vi "Begin.vi"() -> (0 "error out":errorcluster)   [LabVIEW 2011]
doc: "Called before other user functions, this VI is expected to open initial I/O refnums, load in file data, and do all program initialization. Notice that the <B>error out</B> terminal is simply used for data flow. Wiring it to other structures or subVIs ensures that this VI runs first."
uses:
  <vilib>/Rock Robotics/WPI/Joystick/WPI_JoystickDeviceEnum.ctl
  <vilib>/Rock Robotics/SystemInterfaces/AI/FPGA_AIChannel.ctl
  <vilib>/Rock Robotics/SystemInterfaces/Typedef/FPGA_TypedefAnalogModule.ctl
  <vilib>/Rock Robotics/SystemInterfaces/Typedef/FPGA_TypedefDigitalModule.ctl
  <vilib>/Rock Robotics/SystemInterfaces/DIO/FPGA_DIOPWMChannel.ctl
  <vilib>/Rock Robotics/WPI/Relay/WPI_RelayDirection.ctl
  <vilib>/Rock Robotics/SystemInterfaces/DIO/FPGA_DIORelayChannel.ctl
  <vilib>/Rock Robotics/SystemInterfaces/DIO/FPGA_DIOChannel.ctl
  <vilib>/Rock Robotics/WPI/Encoder/WPI_EncoderType.ctl
  <vilib>/Rock Robotics/WPI/MotorControl/WPI_MotorControlOpen Victor.vi
  <vilib>/Rock Robotics/WPI/MotorControl/WPI_MotorControlOpen Jaguar.vi
  Robot Global Data.vi
  <vilib>/Rock Robotics/WPI/Counter/WPI_CounterDigitalInputToDigitalSource.vi
  <vilib>/Rock Robotics/WPI/RobotDrive/WPI_RobotDriveOpen2MotorWithVictor.vi
panel:
  out "Top 45":dbl[](array[numeric])
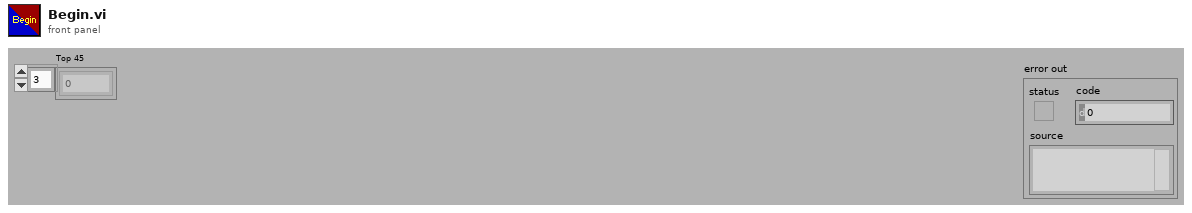
[diagram p1: front panel]
types:
  T1 = typedef "FPGA_DIOPWMChannel.ctl" = enum8{"PWM 1", "PWM 2", "PWM 3", "PWM 4", "PWM 5", "PWM 6", "PWM 7", "PWM 8", "PWM 9", "PWM 10", "Invalid"}
  T2 = typedef "FPGA_TypedefDigitalModule.ctl" = enum16{"Digital Module 1", "Digital Module 2"}
  T3 = enum16{"Shoot", "Load", "Arm", "Nothing", "Reverse", "ShootAll"}
  T4 = typedef "FPGA_DIOChannel.ctl" = enum8{"DIO 1", "DIO 2", "DIO 3", "DIO 4", "DIO 5", "DIO 6", "DIO 7", "DIO 8", "DIO 9", "DIO 10", "DIO 11", "DIO 12", "DIO 13", "DIO 14", "Invalid"}
  T5 = typedef "WPI_EncoderType.ctl" = enum16{"1x", "2x", "4x"}
  T6 = typedef "FPGA_DIORelayChannel.ctl" = enum8{"Relay 1", "Relay 2", "Relay 3", "Relay 4", "Relay 5", "Relay 6", "Relay 7", "Relay 8", "Invalid"}
  T7 = typedef "WPI_RelayDirection.ctl" = enum16{"Both directions", "Forward only", "Reverse only"}
  T8 = typedef "FPGA_TypedefAnalogModule.ctl" = enum16{"Analog Module 1", "Analog Module 2"}
  T9 = typedef "FPGA_AIChannel.ctl" = enum8{"AI 1", "AI 2", "AI 3", "AI 4", "AI 5", "AI 6", "AI 7", "AI 8", "Invalid"}
  T10 = typedef "WPI_JoystickDeviceEnum.ctl" = enum16{"USB 1", "USB 2", "USB 3", "USB 4", "Kinect 1", "Kinect 2"}
  T11 = typedef "FPGA_WatchdogDevRef.ctl" = cluster{"DevStatus":errorcluster}
  T12 = typedef "WPI_RobotDriveDevRef.ctl" = cluster{"DevStatus":errorcluster, "Motors[]":T13[], "Square Inputs":bool, "Max Output":dbl, "Isochronous":bool}
  T13 = typedef "WPI_MotorControlDeviceRef.ctl" = cluster{"DeviceStatus":errorcluster, "Type":enum16{"PWM", "CAN"}, "PWM":cluster{"Digital Module":T2, "PWM Channel":T1, "DeadBand":T14}, "CAN":cluster{"Device Number":u8, "Control Mode":T15, "Semaphore":T16, "Max Vout":dbl}, "Invert":bool, "TransformRef":T17, "InvTransformRef":T17}
  T14 = typedef "WPI_PWMDeadband.ctl" = cluster{"Name":string, "maxPositivePwm":i32, "minPositivePwm":i32, "centerPwm":i32, "maxNegativePwm":i32, "minNegativePwm":i32, "angularRange":u16}
  T15 = typedef "WPI_CANJaguar_ControlMode.ctl" = enum8{"Percent VBus", "Current", "Speed", "Position", "Voltage"}
  T16 = typedef "Semaphore RefNum" = refnum<k1>
  T17 = typedef "WPI_PWMTransform_ConPane.ctl" = refnum<vi>
  T18 = typedef "WPI_JoystickDevRef.ctl" = cluster{"Device":T10}
  T19 = typedef "WPI_AnalogChannelDevRef.ctl" = cluster{"DevStatus":errorcluster, "Analog Module":T8, "Analog Channel":T9}
  T20 = typedef "WPI_DigitalInputDevRef.ctl" = cluster{"DevStatus":errorcluster, "DIO Channel":T4, "Digital Module":T2}
  T21 = typedef "FPGA_CounterEncoderSourceConvertionLVSourceType.ctl" = cluster{"DevStatus":errorcluster, "AnalogTriggerMode?":bool, "DigitalMode":cluster{"Digital Module":T2, "DIO Channel":T22}, "AnalogTriggerMode":cluster{"AnalogTriggerIndex":T23, "OutputType":T24}}
  T22 = typedef "FPGA_DIODigitalSourceChannel.ctl" = enum8{"DIO 1", "DIO 2", "DIO 3", "DIO 4", "DIO 5", "DIO 6", "DIO 7", "DIO 8", "DIO 9", "DIO 10", "DIO 11", "DIO 12", "DIO 13", "DIO 14", "Disabled"}
  T23 = typedef "FPGA_AnalogTriggerIndex.ctl" = enum8{"Trig 0", "Trig 1", "Trig 2", "Trig 3", "Trig 4", "Trig 5", "Trig 6", "Trig 7", "Invalid"}
  T24 = typedef "FPGA_AnalogTriggerOutType.ctl" = enum16{"InWindow", "TriggerState", "Rising", "Falling"}
  T25 = typedef "WPI_EncoderDevRef.ctl" = cluster{"DevStatus":errorcluster, "EncoderIndex":T26, "CounterIndex":T27, "DistancePerCount":dbl, "Decoding Type":T5}
  T26 = typedef "FPGA_EncoderIdx.ctl" = enum8{"Enc 0", "Enc 1", "Enc 2", "Enc 3", "Invalid"}
  T27 = typedef "FPGA_CounterCtrSystemIndex.ctl" = enum8{"Ctr 0", "Ctr 1", "Ctr 2", "Ctr 3", "Ctr 4", "Ctr 5", "Ctr 6", "Ctr 7", "Invalid"}
  T28 = typedef "WPI_RelayDevRef.ctl" = cluster{"DevStatus":errorcluster, "Relay Channel":T6, "Digital Module":T2, "Relay Direction":T7}
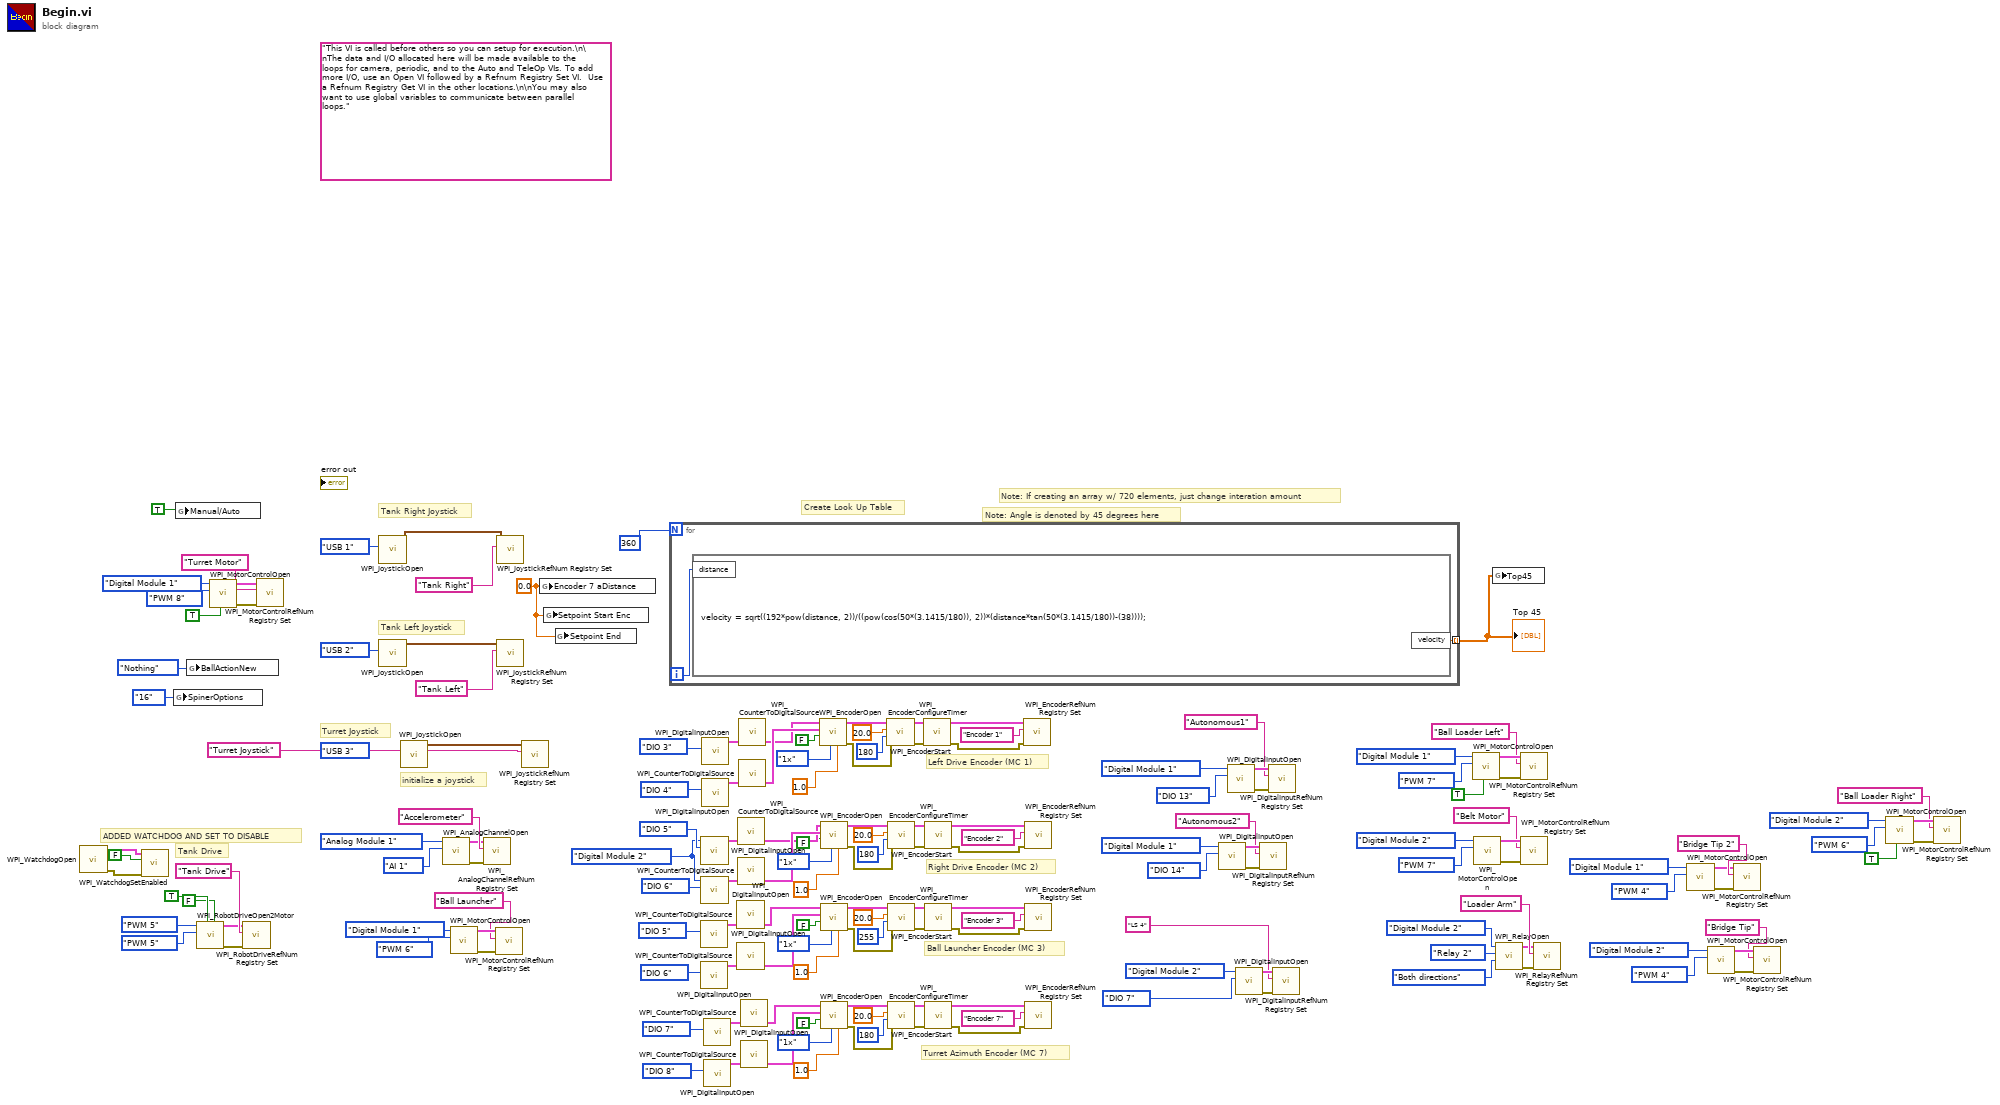
[diagram p0: block diagram]
diagram:
  w29 = FPGA_TypedefDigitalModule."Digital Module 2" ("Digital Module (Module 1)")
  w9 = 0.0 ("Encoder 7 aDistance")
  (unwired) "This VI is called before others so you can setup for execution.\n\nThe data and I/O allocated here will be made available to the loops for camera, periodic, and to the Auto and TeleOp VIs. To add more I/O, use an Open VI followed by a Refnum Registry Set VI.  Use a Refnum Registry Get VI in the other locations.\n\nYou may also want to use global variables to communicate between parallel loops."
  # "Ball Launcher Encoder (MC 3)"
  # "Right Drive Encoder (MC 2)"
  # "Left Drive Encoder (MC 1)"
  # "Tank Drive"
  # "Turret Azimuth Encoder (MC 7)"
  # "ADDED WATCHDOG AND SET TO DISABLE"
  # "Note: Angle is denoted by 45 degrees here"
  # "Note: If creating an array w/ 720 elements, just change interation amount"
  # "Create Look Up Table"
  # "Tank Right Joystick"
  # "Tank Left Joystick"
  # "Turret Joystick"
  # "initialize a joystick"
  n1 = call <vilib>:"WPI_WatchdogOpen.vi"() -> ("error out"=w107:errorcluster, "WatchdogDevRef"=w106:T11)  [unwired: 10 in]
  n2 = call <vilib>:"WPI_WatchdogSetEnabled.vi"("error in (no error)"=w107, "Enabled"=FALSE, "WatchdogDevRef"=w106) -> ()  [unwired: 7 in, 2 out]
  n3 = global write "Robot Global Data.vi" "SpinerOptions"(enum16{"Full", "16", "14", "12", "Poop"}."16" ("SpinerOptions")) -> ()
  n4 = global write "Robot Global Data.vi" "Manual/Auto"(TRUE) -> ()
  n5 = global write "Robot Global Data.vi" "BallActionNew"(T3."Nothing" ("BallActionNew")) -> ()
  n6 = call-poly <vilib>:"WPI_RobotDriveOpen2Motor.vi"("Right Motor Inverted"=FALSE, "Left Motor Inverted"=TRUE, "Right Motor"=FPGA_DIOPWMChannel."PWM 5", "Left Motor"=FPGA_DIOPWMChannel."PWM 5") -> ("error out"=w84:errorcluster, "RobotDriveDevRef"=w82:T12)  [unwired: 6 in]
  n7 = call-poly <vilib>:"WPI_MotorControlOpen.vi"("Invert"=TRUE, "PWM Channel"=FPGA_DIOPWMChannel."PWM 8", "Digital Module (Module 1)"=FPGA_TypedefDigitalModule."Digital Module 1") -> ("error out"=w122:errorcluster, "MotorControlDeviceRef"=w121:T13)  [unwired: 7 in]
  n8 = call <vilib>:"WPI_RobotDriveRefNum Registry Set.vi"("error in (no error)"=w84, "refnum name"="Tank Drive", "RobotDriveDevRef"=w82) -> ()  [unwired: 7 in, 2 out]
  n9 = call <vilib>:"WPI_MotorControlRefNum Registry Set.vi"("error in (no error)"=w122, "refnum name"="Turret Motor", "MotorControlDevRef"=w121) -> ()  [unwired: 7 in, 2 out]
  n10 = call <vilib>:"WPI_JoystickOpen.vi"("JoystickDevice"=WPI_JoystickDeviceEnum."USB 1") -> ("JoystickDevRef"=w156:T18)  [unwired: 10 in]
  n11 = call <vilib>:"WPI_JoystickOpen.vi"("JoystickDevice"=WPI_JoystickDeviceEnum."USB 2") -> ("JoystickDevRef"=w159:T18)  [unwired: 10 in]
  n12 = call <vilib>:"WPI_JoystickOpen.vi"("JoystickDevice"=WPI_JoystickDeviceEnum."USB 3") -> ("JoystickDevRef"=w162:T18)  [unwired: 10 out]
  n13 = call <vilib>:"WPI_AnalogChannelOpen.vi"("Analog Channel"=FPGA_AIChannel."AI 1", "Analog Module (Module 1)"=FPGA_TypedefAnalogModule."Analog Module 1") -> ("error out"=w151:errorcluster, "AIDeviceRef"=w152:T19)  [unwired: 8 in]
  n14 = call-poly <vilib>:"WPI_MotorControlOpen.vi"("PWM Channel"=FPGA_DIOPWMChannel."PWM 6", "Digital Module (Module 1)"=FPGA_TypedefDigitalModule."Digital Module 1") -> ("error out"=w148:errorcluster, "MotorControlDeviceRef"=w147:T13)  [unwired: 8 in]
  n15 = call <vilib>:"WPI_AnalogChannelRefNum Registry Set.vi"("error in (no error)"=w151, "refnum name"="Accelerometer", "AIDeviceRef"=w152) -> ()  [unwired: 7 in, 2 out]
  n16 = call <vilib>:"WPI_MotorControlRefNum Registry Set.vi"("error in (no error)"=w148, "refnum name"="Ball Launcher", "MotorControlDevRef"=w147) -> ()  [unwired: 7 in, 2 out]
  n17 = call <vilib>:"WPI_JoystickRefNum Registry Set.vi"("refnum name"="Tank Right", "JoystickDevRef"=w156) -> ()  [unwired: 8 in, 2 out]
  n18 = call <vilib>:"WPI_JoystickRefNum Registry Set.vi"("refnum name"="Tank Left", "JoystickDevRef"=w159) -> ()  [unwired: 8 in, 2 out]
  n19 = call <vilib>:"WPI_JoystickRefNum Registry Set.vi"("refnum name"="Turret Joystick", "JoystickDevRef"=w162) -> ()  [unwired: 1 in, 9 out]
  n20 = global write "Robot Global Data.vi" "Encoder 7 aDistance"(w9) -> ()
  n21 = global write "Robot Global Data.vi" "Setpoint Start Enc"(w9) -> ()
  n22 = global write "Robot Global Data.vi" "Setpoint End"(w9) -> ()
  n23 = for {
    N: 360 -> [_]
    tunnel: [w163] -> w108 mode=indexing
    i -> [w164]
    n24 = formula code="velocity = sqrt((192*pow(distance, 2))/((pow(cos(50*(3.1415/180)), 2))*(distance*tan(50*(3.1415/180))-(38))));"("distance"=w164) -> ("velocity"=w163:dbl)
  }
  "Top 45" <- w108
  n25 = call <vilib>:"WPI_DigitalInputOpen.vi"("DIO Channel"=FPGA_DIOChannel."DIO 5") -> ("DigitalInputDevRef"=w42:T20)  [unwired: 2 in, 8 out]
  n26 = call <vilib>:"WPI_DigitalInputOpen.vi"("DIO Channel"=FPGA_DIOChannel."DIO 6") -> ("DigitalInputDevRef"=w43:T20)  [unwired: 2 in, 8 out]
  n27 = call <vilib>:"WPI_DigitalInputOpen.vi"("DIO Channel"=FPGA_DIOChannel."DIO 5", "Digital Module (Module 1)"=w29) -> ("DigitalInputDevRef"=w57:T20)  [unwired: 1 in, 8 out]
  n28 = call <vilib>:"WPI_DigitalInputOpen.vi"("DIO Channel"=FPGA_DIOChannel."DIO 6", "Digital Module (Module 1)"=w29) -> ("DigitalInputDevRef"=w58:T20)  [unwired: 1 in, 8 out]
  n29 = call <vilib>:"WPI_DigitalInputOpen.vi"("DIO Channel"=FPGA_DIOChannel."DIO 3") -> ("DigitalInputDevRef"=w72:T20)  [unwired: 2 in, 8 out]
  n30 = call <vilib>:"WPI_DigitalInputOpen.vi"("DIO Channel"=FPGA_DIOChannel."DIO 4") -> ("DigitalInputDevRef"=w73:T20)  [unwired: 2 in, 8 out]
  n31 = call <vilib>:"WPI_DigitalInputOpen.vi"("DIO Channel"=FPGA_DIOChannel."DIO 7") -> ("DigitalInputDevRef"=w102:T20)  [unwired: 2 in, 8 out]
  n32 = call <vilib>:"WPI_DigitalInputOpen.vi"("DIO Channel"=FPGA_DIOChannel."DIO 8") -> ("DigitalInputDevRef"=w103:T20)  [unwired: 2 in, 8 out]
  n33 = call-poly <vilib>:"WPI_CounterToDigitalSource.vi"("DigitalInputDevRef"=w42) -> ("Digital Source"=w41:T21)  [unwired: 6 out]
  n34 = call-poly <vilib>:"WPI_CounterToDigitalSource.vi"("DigitalInputDevRef"=w43) -> ("Digital Source"=w44:T21)  [unwired: 6 out]
  n35 = call-poly <vilib>:"WPI_CounterToDigitalSource.vi"("DigitalInputDevRef"=w57) -> ("Digital Source"=w56:T21)  [unwired: 6 out]
  n36 = call-poly <vilib>:"WPI_CounterToDigitalSource.vi"("DigitalInputDevRef"=w58) -> ("Digital Source"=w59:T21)  [unwired: 6 out]
  n37 = call-poly <vilib>:"WPI_CounterToDigitalSource.vi"("DigitalInputDevRef"=w72) -> ("Digital Source"=w71:T21)  [unwired: 6 out]
  n38 = call-poly <vilib>:"WPI_CounterToDigitalSource.vi"("DigitalInputDevRef"=w73) -> ("Digital Source"=w74:T21)  [unwired: 6 out]
  n39 = call-poly <vilib>:"WPI_CounterToDigitalSource.vi"("DigitalInputDevRef"=w102) -> ("Digital Source"=w101:T21)  [unwired: 6 out]
  n40 = call-poly <vilib>:"WPI_CounterToDigitalSource.vi"("DigitalInputDevRef"=w103) -> ("Digital Source"=w104:T21)  [unwired: 6 out]
  n41 = call <vilib>:"WPI_EncoderOpen.vi"("DistancePerCount"=1.0, "Decoding Type"=WPI_EncoderType."1x", "Invert Direction (False)"=FALSE ("Invert Direction"), "BSource"=w74, "ASource"=w71) -> ("error out"=w25:errorcluster, "EncoderDevRef"=w66:T25)  [unwired: 3 in, 2 out]
  n42 = call <vilib>:"WPI_EncoderOpen.vi"("DistancePerCount"=1.0, "Decoding Type"=WPI_EncoderType."1x", "Invert Direction (False)"=FALSE ("Invert Direction"), "BSource"=w59, "ASource"=w56) -> ("error out"=w24:errorcluster, "EncoderDevRef"=w51:T25)  [unwired: 3 in, 2 out]
  n43 = call <vilib>:"WPI_EncoderOpen.vi"("DistancePerCount"=1.0, "Decoding Type"=WPI_EncoderType."1x", "Invert Direction (False)"=FALSE ("Invert Direction"), "BSource"=w44, "ASource"=w41) -> ("error out"=w23:errorcluster, "EncoderDevRef"=w36:T25)  [unwired: 3 in, 2 out]
  n44 = call <vilib>:"WPI_EncoderOpen.vi"("DistancePerCount"=1.0, "Decoding Type"=WPI_EncoderType."1x", "Invert Direction (False)"=FALSE ("Invert Direction"), "BSource"=w104, "ASource"=w101) -> ("error out"=w76:errorcluster, "EncoderDevRef"=w96:T25)  [unwired: 3 in, 2 out]
  n45 = call <vilib>:"WPI_EncoderConfigureTimer.vi"("error in (no error)"=w25, "Number Samples to Average"=u8 180, "Minimum Rate"=20.0, "EncoderDevRef"=w66) -> ("error out"=w26:errorcluster, "EncoderDevRef"=w67:T25)  [unwired: 6 out]
  n46 = call <vilib>:"WPI_EncoderConfigureTimer.vi"("error in (no error)"=w24, "Number Samples to Average"=u8 180, "Minimum Rate"=20.0, "EncoderDevRef"=w51) -> ("error out"=w27:errorcluster, "EncoderDevRef"=w52:T25)  [unwired: 6 out]
  n47 = call <vilib>:"WPI_EncoderConfigureTimer.vi"("error in (no error)"=w23, "Number Samples to Average"=u8 255, "Minimum Rate"=20.0, "EncoderDevRef"=w36) -> ("error out"=w28:errorcluster, "EncoderDevRef"=w37:T25)  [unwired: 6 out]
  n48 = call <vilib>:"WPI_EncoderConfigureTimer.vi"("error in (no error)"=w76, "Number Samples to Average"=u8 180, "Minimum Rate"=20.0, "EncoderDevRef"=w96) -> ("error out"=w77:errorcluster, "EncoderDevRef"=w97:T25)  [unwired: 6 out]
  n49 = call <vilib>:"WPI_EncoderStart.vi"("error in (no error)"=w26, "EncoderDevRef"=w67) -> ("error out"=w20:errorcluster, "EncoderDevRef"=w63:T25)  [unwired: 8 out]
  n50 = call <vilib>:"WPI_EncoderStart.vi"("error in (no error)"=w27, "EncoderDevRef"=w52) -> ("error out"=w21:errorcluster, "EncoderDevRef"=w48:T25)  [unwired: 8 out]
  n51 = call <vilib>:"WPI_EncoderStart.vi"("error in (no error)"=w28, "EncoderDevRef"=w37) -> ("error out"=w22:errorcluster, "EncoderDevRef"=w33:T25)  [unwired: 8 out]
  n52 = call <vilib>:"WPI_EncoderStart.vi"("error in (no error)"=w77, "EncoderDevRef"=w97) -> ("error out"=w75:errorcluster, "EncoderDevRef"=w93:T25)  [unwired: 8 out]
  n53 = call <vilib>:"WPI_EncoderRefNum Registry Set.vi"("error in (no error)"=w20, "refnum name"="Encoder 1", "EncoderDevRef"=w63) -> ()  [unwired: 7 in, 2 out]
  n54 = call <vilib>:"WPI_EncoderRefNum Registry Set.vi"("error in (no error)"=w21, "refnum name"="Encoder 2", "EncoderDevRef"=w48) -> ()  [unwired: 7 in, 2 out]
  n55 = call <vilib>:"WPI_EncoderRefNum Registry Set.vi"("error in (no error)"=w22, "refnum name"="Encoder 3", "EncoderDevRef"=w33) -> ()  [unwired: 7 in, 2 out]
  n56 = call <vilib>:"WPI_EncoderRefNum Registry Set.vi"("error in (no error)"=w75, "refnum name"="Encoder 7", "EncoderDevRef"=w93) -> ()  [unwired: 7 in, 2 out]
  n57 = call <vilib>:"WPI_DigitalInputOpen.vi"("DIO Channel"=FPGA_DIOChannel."DIO 14", "Digital Module (Module 1)"=FPGA_TypedefDigitalModule."Digital Module 1") -> ("error out"=w12:errorcluster, "DigitalInputDevRef"=w13:T20)  [unwired: 8 in]
  n58 = call <vilib>:"WPI_DigitalInputOpen.vi"("DIO Channel"=FPGA_DIOChannel."DIO 13", "Digital Module (Module 1)"=FPGA_TypedefDigitalModule."Digital Module 1") -> ("error out"=w19:errorcluster, "DigitalInputDevRef"=w18:T20)  [unwired: 8 in]
  n59 = call <vilib>:"WPI_DigitalInputOpen.vi"("DIO Channel"=FPGA_DIOChannel."DIO 7", "Digital Module (Module 1)"=FPGA_TypedefDigitalModule."Digital Module 2") -> ("error out"=w87:errorcluster, "DigitalInputDevRef"=w86:T20)  [unwired: 8 in]
  n60 = call <vilib>:"WPI_DigitalInputRefNum Registry Set.vi"("error in (no error)"=w12, "refnum name"="Autonomous2", "DigitalInputDevRef"=w13) -> ()  [unwired: 7 in, 2 out]
  n61 = call <vilib>:"WPI_DigitalInputRefNum Registry Set.vi"("error in (no error)"=w19, "refnum name"="Autonomous1", "DigitalInputDevRef"=w18) -> ()  [unwired: 7 in, 2 out]
  n62 = call <vilib>:"WPI_DigitalInputRefNum Registry Set.vi"("error in (no error)"=w87, "refnum name"="LS 4", "DigitalInputDevRef"=w86) -> ()  [unwired: 7 in, 2 out]
  n63 = call-poly <vilib>:"WPI_MotorControlOpen.vi"("Invert"=TRUE, "PWM Channel"=FPGA_DIOPWMChannel."PWM 7", "Digital Module (Module 1)"=FPGA_TypedefDigitalModule."Digital Module 1") -> ("error out"=w143:errorcluster, "MotorControlDeviceRef"=w142:T13)  [unwired: 7 in]
  n64 = call-poly <vilib>:"WPI_MotorControlOpen.vi"("PWM Channel"=FPGA_DIOPWMChannel."PWM 7", "Digital Module (Module 1)"=FPGA_TypedefDigitalModule."Digital Module 2") -> ("error out"=w137:errorcluster, "MotorControlDeviceRef"=w136:T13)  [unwired: 8 in]
  n65 = global write "Robot Global Data.vi" "Top45"(w108) -> ()
  n66 = call <vilib>:"WPI_RelayOpen.vi"("Relay Direction"=WPI_RelayDirection."Both directions", "Relay Channel"=FPGA_DIORelayChannel."Relay 2", "Digital Module (Module 1)"=FPGA_TypedefDigitalModule."Digital Module 2") -> ("error out"=w110:errorcluster, "RelayDevRef"=w111:T28)  [unwired: 7 in]
  n67 = call <vilib>:"WPI_MotorControlRefNum Registry Set.vi"("error in (no error)"=w143, "refnum name"="Ball Loader Left", "MotorControlDevRef"=w142) -> ()  [unwired: 7 in, 2 out]
  n68 = call <vilib>:"WPI_MotorControlRefNum Registry Set.vi"("error in (no error)"=w137, "refnum name"="Belt Motor", "MotorControlDevRef"=w136) -> ()  [unwired: 7 in, 2 out]
  n69 = call <vilib>:"WPI_RelayRefNum Registry Set.vi"("error in (no error)"=w110, "refnum name"="Loader Arm", "RelayDevRef"=w111) -> ()  [unwired: 7 in, 2 out]
  n70 = call-poly <vilib>:"WPI_MotorControlOpen.vi"("PWM Channel"=FPGA_DIOPWMChannel."PWM 4", "Digital Module (Module 1)"=FPGA_TypedefDigitalModule."Digital Module 1") -> ("error out"=w2:errorcluster, "MotorControlDeviceRef"=w3:T13)  [unwired: 8 in]
  n71 = call-poly <vilib>:"WPI_MotorControlOpen.vi"("PWM Channel"=FPGA_DIOPWMChannel."PWM 4", "Digital Module (Module 1)"=FPGA_TypedefDigitalModule."Digital Module 2") -> ("error out"=w116:errorcluster, "MotorControlDeviceRef"=w115:T13)  [unwired: 8 in]
  n72 = call <vilib>:"WPI_MotorControlRefNum Registry Set.vi"("error in (no error)"=w2, "refnum name"="Bridge Tip 2", "MotorControlDevRef"=w3) -> ()  [unwired: 7 in, 2 out]
  n73 = call <vilib>:"WPI_MotorControlRefNum Registry Set.vi"("error in (no error)"=w116, "refnum name"="Bridge Tip", "MotorControlDevRef"=w115) -> ()  [unwired: 7 in, 2 out]
  n74 = call-poly <vilib>:"WPI_MotorControlOpen.vi"("Invert"=TRUE, "PWM Channel"=FPGA_DIOPWMChannel."PWM 6", "Digital Module (Module 1)"=FPGA_TypedefDigitalModule."Digital Module 2") -> ("error out"=w140:errorcluster, "MotorControlDeviceRef"=w139:T13)  [unwired: 7 in]
  n75 = call <vilib>:"WPI_MotorControlRefNum Registry Set.vi"("error in (no error)"=w140, "refnum name"="Ball Loader Right", "MotorControlDevRef"=w139) -> ()  [unwired: 7 in, 2 out]
